vi "calibrate RP.vi"() -> ()   [LabVIEW 2018]
uses:
  Libraries/Instruments/Pulse Driver/Pusle Driver Configuration.ctl
  Libraries/Red Pitaya/RP EEPROM Calibration.ctl
  Libraries/Red Pitaya/Red Pitaya Digitizer/Red Pitaya Digitizer.lvclass
  C:/github/NHMFL_Core/Libraries/Instruments/Pulse Driver/Pulse Driver.lvclass
  Libraries/Red Pitaya/Red Pitaya Digitizer/Write Server address.vi
panel:
  in  "Copy":bool
  in  "Trial calibration":T1={"In1 LV scale"=49836223, "In2 LV scale"=49694489, "In1 HV scale"=896952379, "In2 HV scale"=896565832, "In1 HV offset"=-101, "In2 HV offset"=-51, "Out1 scale"=42827309, "Out2 scale"=43127055, "Out1 offset"=-40, "Out2 offset"=-40, "magic"=2864434397, "In1 LV offset"=-136, "In2 LV offset"=-62} {"magic" format="%x"}
  out "Server  output":string
  in  "Write calib":bool
  in  "calib parameters":string
  in  "Read calib":bool
  out "Mean (DC)":dbl[](array[numeric])
  out "Peak to Peak":dbl[](array[numeric])
  out "RP EEPROM Calibration":T1 {"magic" format="%x"}
  in  "milliseconds to wait":u32=100
  out "Waveform Graph":dbl[][](graph)
  in  "RP address":string="192.168.1.100"
  in  "Pulse Configuration":T2={"Pre-trigger duration"=0.001, "Post-trigger duration"=0.001, "Rate"=125000000.0, "Ranges"=[1.0, 1.0], "Re-name channels"=[], "Active channels"="0:1", "External clock"=FALSE} {"Rate" format="%#_8pHz"; "Post-trigger duration" format="%#_6ps"; "Pre-trigger duration" format="%#_6ps"; "Ranges" format="%#_6pV"}
  in  "Read data":bool
  in  "stop":bool
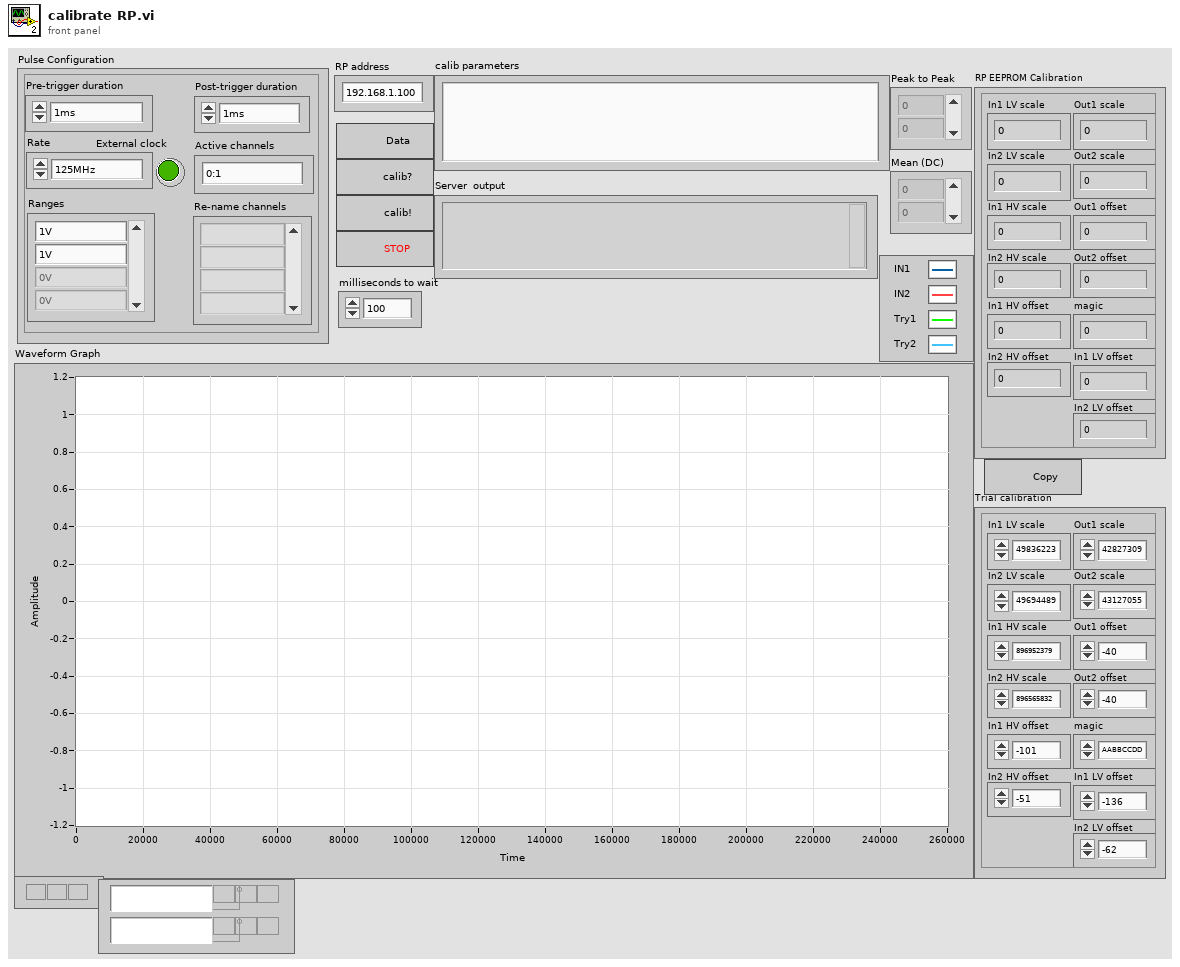
[diagram p1: front panel]
types:
  T1 = typedef "RP EEPROM Calibration.ctl" = cluster{"In1 LV scale":u32, "In2 LV scale":u32, "In1 HV scale":u32, "In2 HV scale":u32, "In1 HV offset":i32, "In2 HV offset":i32, "Out1 scale":u32, "Out2 scale":u32, "Out1 offset":i32, "Out2 offset":i32, "magic":u32, "In1 LV offset":i32, "In2 LV offset":i32}
  T2 = typedef "Pusle Driver Configuration.ctl" = cluster{"Pre-trigger duration":dbl, "Post-trigger duration":dbl, "Rate":dbl, "Ranges":dbl[], "Re-name channels":string[], "Active channels":string, "External clock":bool}
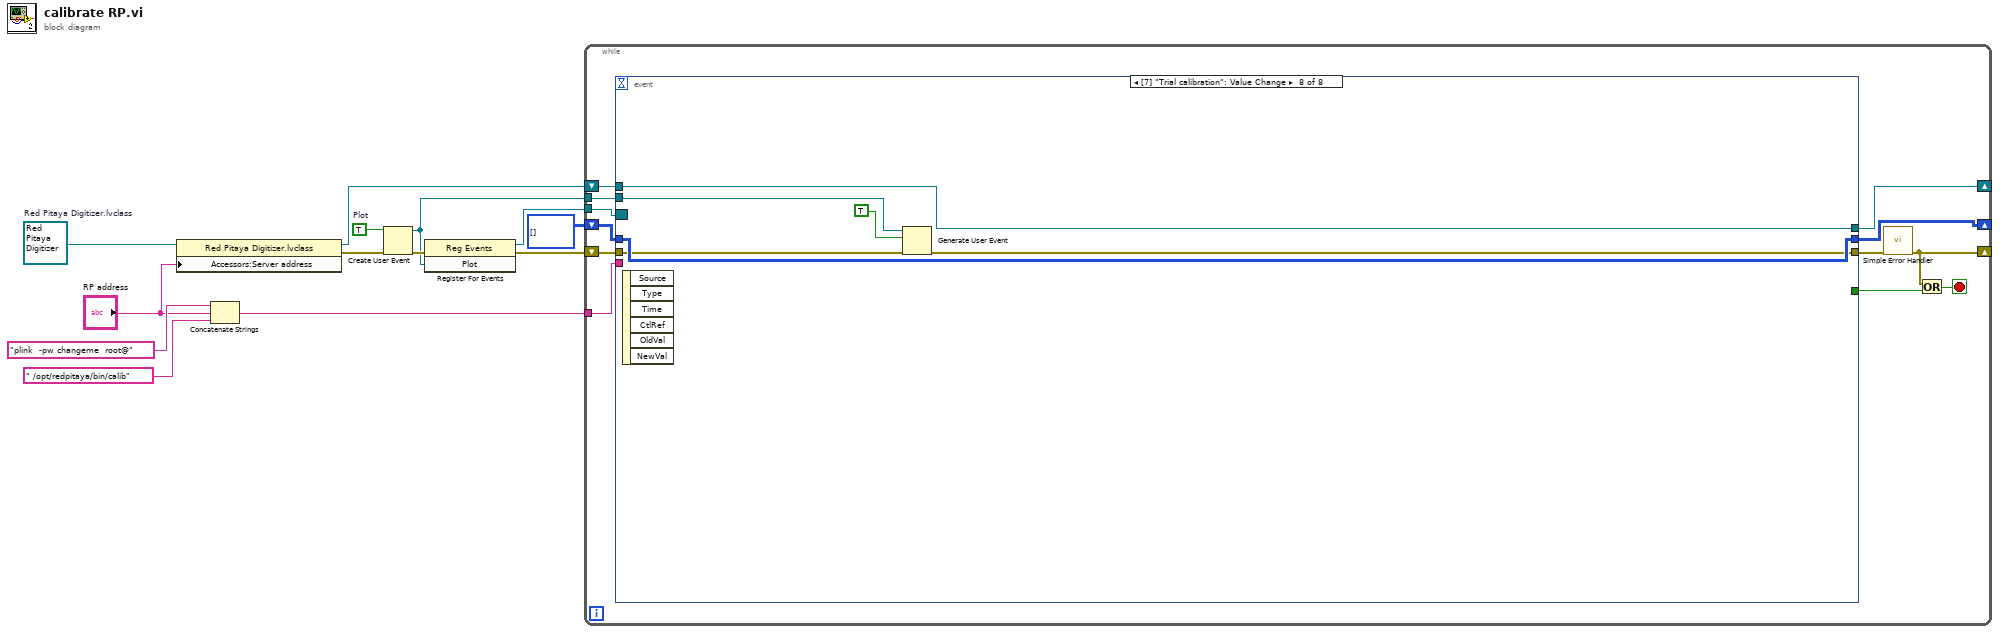
[diagram p0: block diagram]
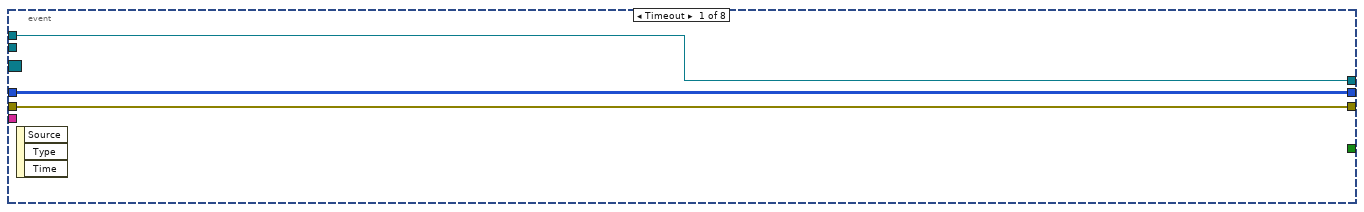
[diagram p2: hidden frame]
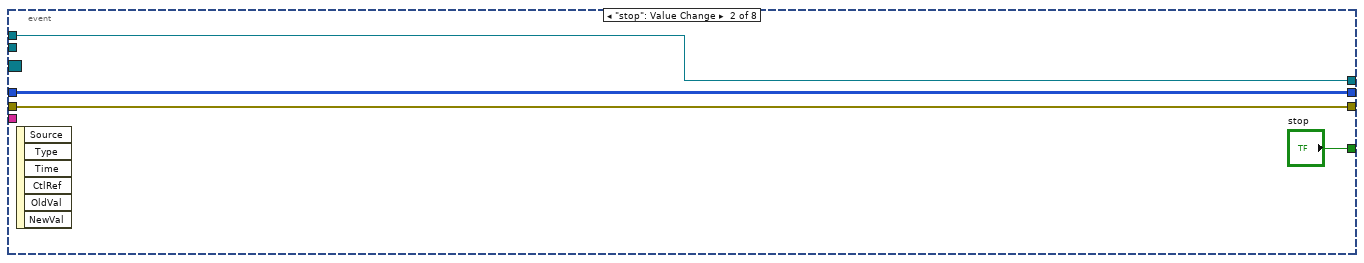
[diagram p3: hidden frame]
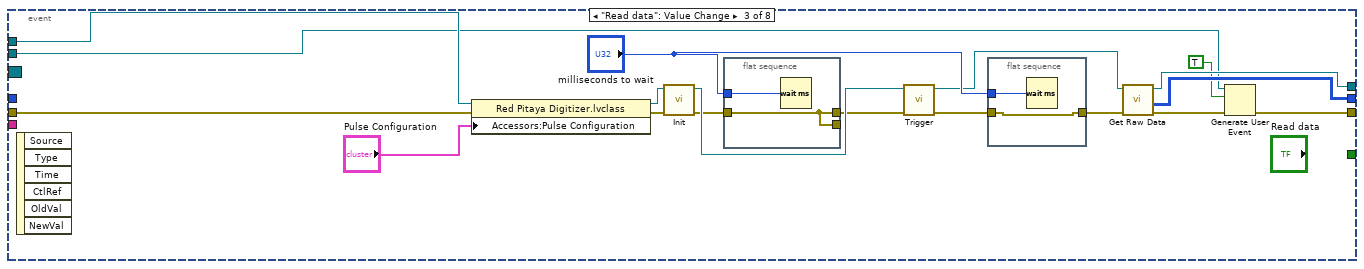
[diagram p4: hidden frame]
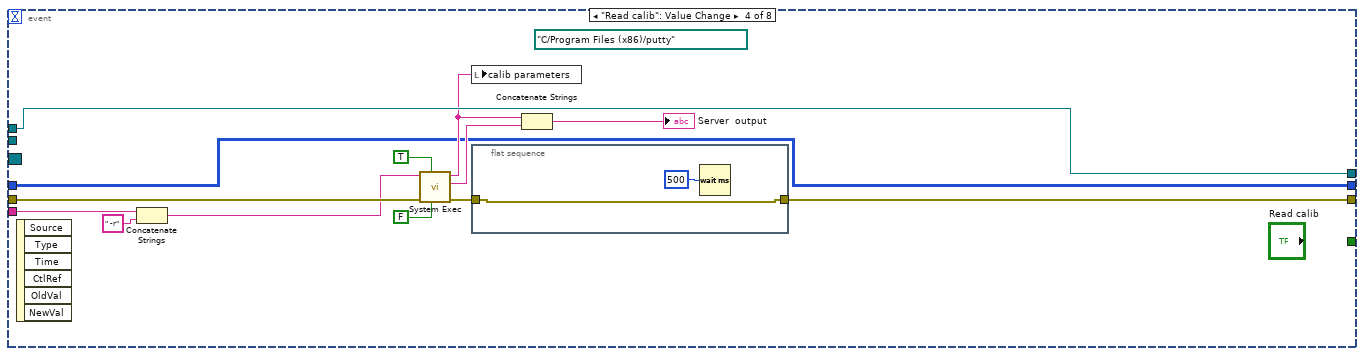
[diagram p5: hidden frame]
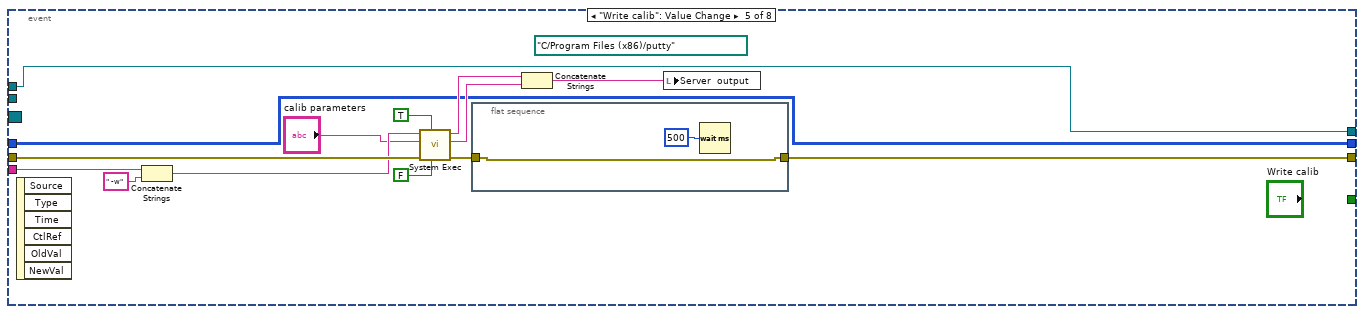
[diagram p6: hidden frame]
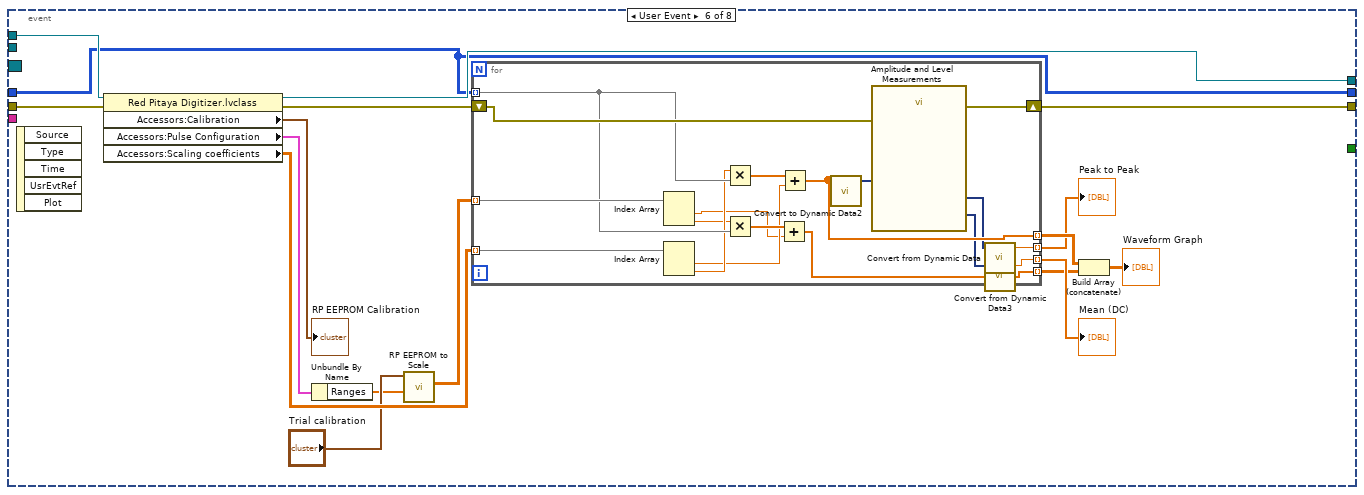
[diagram p7: hidden frame]
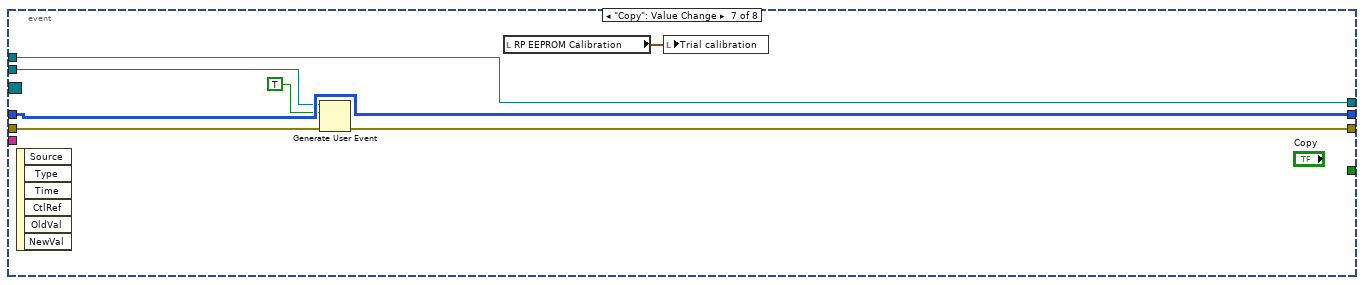
[diagram p8: hidden frame]
diagram:
  w7 = TRUE  # Plot
  w13 = refnum<class "Red Pitaya Digitizer.lvclass"> refnum  # Red Pitaya Digitizer.lvclass
  n1 = property class="Red Pitaya Digitizer.lvclass"(reference=w13, "Accessors:Server address"="RP address") -> (reference out=w12:refnum<class "Red Pitaya Digitizer.lvclass">, error out=w6:errorcluster)  [unwired: 1 in]
  n2 = Concatenate Strings("plink  -pw changeme  root@" ("command line"), "RP address", " /opt/redpitaya/bin/calib" ("command line")) -> (w8:string)
  n3 = Create User Event(user event datatype=w7, error in=w6) -> (user event=w1:refnum<user-event>, error out=w4:errorcluster)
  n4 = register-events(error in=w4, w1) -> (reference out=w5:refnum<event-registration>, error out=w3:errorcluster)  [unwired: 1 in]
  n5 = while {
    shift-right: [w21] -> _
    shift-left: w12 -> [w24]
    shift-right: [w19] -> _
    shift-left: w3 -> [w22]
    tunnel: w8 -> [w18]
    tunnel: w5 -> [w17]
    shift-right: [w16] -> _
    shift-left: i16[][] [] ("appended array") -> [w15]
    tunnel: w1 -> [w14]
    stop <- w20 stop-if-true
    n6 = event shown="[7] \"Trial calibration\": Value Change" {
      selector: w17 -> [_ _ _ _ _ _ _ _]
      dyn-events: _ -> [_ _ _ _ _ _ _ _]
      timeout: _ -> [_ _ _ _ _ _ _ _]
      tunnel: [_ "stop" _ _ _ _ _ _] -> w25
      tunnel: w24 -> [w28 w31 w50 w62 w79 w102 w125 w132]
      tunnel: [w27 w30 w34 w61 w78 w94 w123 w130] -> w23
      tunnel: w22 -> [w27 w30 w45 w63 w80 w101 w122 w129]
      tunnel: [w28 w31 w44 w62 w79 w100 w125 w132] -> w21
      tunnel: w18 -> [_ _ _ w60 w77 _ _ _]
      tunnel: [w26 w29 w39 w55 w70 w98 w126 w133] -> w16
      tunnel: w15 -> [w26 w29 _ w55 w70 w98 w126 w133]
      tunnel: w14 -> [_ _ w36 _ _ _ w121 w128]
      event Timeout {
        n7 = event-data() -> ()  [unwired: 1 in, 3 out]
      }
      event "stop": Value Change {
        n8 = event-data() -> ()  [unwired: 1 in, 6 out]
      }
      event "Read data": Value Change {
        n9 = event-data() -> ()  [unwired: 1 in, 6 out]
        n10 = property class="Red Pitaya Digitizer.lvclass"(reference=w50, error in=w45, "Accessors:Pulse Configuration"="Pulse Configuration") -> (reference out=w48:refnum<class "Red Pitaya Digitizer.lvclass">, error out=w46:errorcluster)
        n11 = call-dynamic "Init.vi"("error in (no error)"=w46, "Instrument Driver in"=w48) -> ("error out"=w41:errorcluster, "Instrument Driver out"=w47:refnum<class "Red Pitaya Digitizer.lvclass">)  [unwired: 7 in, 1 out]
        n12 = flat-sequence {
          tunnel: w41 -> [w51]
          tunnel: [w51] -> _
          tunnel: "milliseconds to wait" -> [w52]
          tunnel: [w51] -> w40
          frame #0 {
            n13 = Wait (ms)(milliseconds to wait=w52) -> ()  [unwired: 1 out]
          }
        }
        n14 = call-dynamic "Trigger.vi"("error in (no error)"=w40, "Red Pitaya Digitizer in"=w47) -> ("error out"=w43:errorcluster, "Red Pitaya Digitizer out"=w38:refnum<class "Red Pitaya Digitizer.lvclass">)  [unwired: 8 in]
        n15 = flat-sequence {
          tunnel: w43 -> [w54]
          tunnel: [w54] -> w37
          tunnel: "milliseconds to wait" -> [w53]
          frame #0 {
            n16 = Wait (ms)(milliseconds to wait=w53) -> ()  [unwired: 1 out]
          }
        }
        n17 = call-dynamic "Get Raw Data.vi"("error in (no error)"=w37, "Red Pitaya Digitizer in"=w38) -> ("error out"=w35:errorcluster, "appended array"=w39:i16[][], "Red Pitaya Digitizer out"=w44:refnum<class "Red Pitaya Digitizer.lvclass">)  [unwired: 7 in]
        n18 = Generate User Event(user event=w36, event data cluster=TRUE ("event data"), error in=w35) -> (error out=w34:errorcluster)  [unwired: 1 in, 1 out]
      }
      event "Read calib": Value Change {
        (unwired) path "C:/Program Files (x86)/putty" ("working directory")
        n19 = event-data() -> ()  [unwired: 1 in, 6 out]
        n20 = Concatenate Strings(w60, " -r" ("string")) -> (w58:string)
        n21 = call <vilib>:"System Exec.vi"("run minimized? (F)"=FALSE, "wait until completion? (T)"=TRUE, "error in (no error)"=w63, "command line"=w58) -> ("error out"=w64:errorcluster, "standard error"=w66:string, "standard output"=w57:string)  [unwired: 4 in, 1 out]
        n22 = local write "calib parameters"(w57) -> ()
        n23 = flat-sequence {
          tunnel: w64 -> [w69]
          tunnel: [w69] -> w61
          frame #0 {
            n24 = Wait (ms)(milliseconds to wait=u32 500) -> ()  [unwired: 1 out]
          }
        }
        n25 = Concatenate Strings(w57, w66) -> (→"Server  output":string)
      }
      event "Write calib": Value Change {
        (unwired) path "C:/Program Files (x86)/putty" ("working directory")
        n26 = event-data() -> ()  [unwired: 1 in, 6 out]
        n27 = Concatenate Strings(w77, " -w" ("string")) -> (w75:string)
        n28 = call <vilib>:"System Exec.vi"("run minimized? (F)"=FALSE, "wait until completion? (T)"=TRUE, "error in (no error)"=w80, "standard input"="calib parameters", "command line"=w75) -> ("error out"=w81:errorcluster, "standard error"=w83:string, "standard output"=w74:string)  [unwired: 3 in, 1 out]
        n29 = flat-sequence {
          tunnel: w81 -> [w85]
          tunnel: [w85] -> w78
          frame #0 {
            n30 = Wait (ms)(milliseconds to wait=u32 500) -> ()  [unwired: 1 out]
          }
        }
        n31 = Concatenate Strings(w74, w83) -> (w72:string)
        n32 = local write "Server  output"(w72) -> ()
      }
      event User Event {
        n33 = event-data() -> ()  [unwired: 1 in, 5 out]
        n34 = property class="Red Pitaya Digitizer.lvclass"(reference=w102, error in=w101) -> (reference out=w100:refnum<class "Red Pitaya Digitizer.lvclass">, error out=w95:errorcluster, "Accessors:Calibration"=→"RP EEPROM Calibration":T1, "Accessors:Pulse Configuration"=w87:T2, "Accessors:Scaling coefficients"=w97:dbl[][])
        n35 = Unbundle By Name(w87) -> ("Ranges"=w86:dbl[])
        n36 = call "RP EEPROM to Scale.vi"("Ranges"=w86, "EEPROM calibration"="Trial calibration") -> ("Scaling coefficients"=w90:dbl[][])  [unwired: 8 in, 1 out]
        n37 = for {
          tunnel: w98 -> [w109] mode=indexing
          tunnel: w97 -> [w120] mode=indexing
          tunnel: [w115] -> w96 mode=indexing
          tunnel: [w113] -> w93 mode=indexing
          tunnel: [w111] -> w92 mode=indexing
          shift-right: [w117] -> w94
          shift-left: w95 -> [w118]
          tunnel: w90 -> [w110] mode=indexing
          tunnel: [w107] -> w88 mode=indexing
          n38 = Index Array(array=w110) -> (element #1=w104:dbl, element #2=w103:dbl)  [unwired: 2 in]
          n39 = Index Array(array=w120) -> (element #1=w105:dbl, element #2=w106:dbl)  [unwired: 2 in]
          n40 = Multiply(x=w106, y=w109) -> (x*y=w119:dbl[])
          n41 = Multiply(x=w103, y=w109) -> (x*y=w108:dbl[])
          n42 = Add(x=w108, y=w104) -> (x+y=w107:dbl[])
          n43 = Add(x=w119, y=w105) -> (x+y=w115:dbl[])
          n44 = call "Convert to Dynamic Data2"("Array"=w115) -> ("Dynamic Data Type"=w116:dynamicdata)  [unwired: 3 in]
          n45 = call "Amplitude and Level Measurements"("Signals"=w116, "error in (no error)"=w118) -> ("Mean (DC)"=w112:dynamicdata, "Peak to Peak"=w114:dynamicdata, "error out"=w117:errorcluster)  [unwired: 11 in]
          n46 = call "Convert from Dynamic Data"("Dynamic Data Type"=w114) -> ("Scalar"=w113:dbl)  [unwired: 3 in]
          n47 = call "Convert from Dynamic Data3"("Dynamic Data Type"=w112) -> ("Scalar"=w111:dbl)  [unwired: 3 in]
        }
        "Peak to Peak" <- w93
        "Mean (DC)" <- w92
        n48 = Build Array (concatenate)(w96, w88) -> (→"Waveform Graph":dbl[][])
      }
      event "Copy": Value Change {
        n49 = event-data() -> ()  [unwired: 1 in, 6 out]
        n50 = Generate User Event(user event=w121, event data cluster=TRUE ("event data"), error in=w122) -> (error out=w123:errorcluster)  [unwired: 1 in, 1 out]
        n51 = local read "RP EEPROM Calibration"() -> (w127:T1)
        n52 = local write "Trial calibration"(w127) -> ()
      }
      event Value Change {
        n53 = event-data() -> ()  [unwired: 1 in, 6 out]
        n54 = Generate User Event(user event=w128, event data cluster=TRUE ("event data"), error in=w129) -> (error out=w130:errorcluster)  [unwired: 1 in, 1 out]
      }
    }
    n55 = call <vilib>:"Simple Error Handler.vi"("error in (no error)"=w23) -> ("error out"=w19:errorcluster)  [unwired: 4 in, 4 out]
    n56 = Or(x=w19, y=w25) -> (x .or. y?=w20:bool)
  }
